vi "Dashboard Main.vi"() -> ()   [LabVIEW 2020]
uses:
  <vilib>/Utility/miscctls.llb/LVRowAndColumnTypeDef.ctl
  <vilib>/event_ctls.llb/eventvkey.ctl
  <vilib>/Rock Robotics/Network Tables/NT Read Numeric Array.vi
  <vilib>/Rock Robotics/WPI/Dashboard/WPI_DashboardLogging Global.vi
panel:
  out "x":dbl(slide) scale=-1.0..1.0 scale format="%#_2e"
  in  "Camera Settings Right":T1={"Frame Rate"=30, "Compression"=30, "Size"=1, "DB Camera Config"=FALSE} {"Frame Rate" scale=1.0..30.0; "Compression" scale=100.0..-1.0; "Size" items=["640x480", "320x240", "160x120"]}
  in  "Camera Name Right":string(combo)="No Camera Selection"
  out "Camera Perf":string
  in  "Camera Settings":T1={"Frame Rate"=30, "Compression"=30, "Size"=1, "DB Camera Config"=FALSE} {"Frame Rate" scale=1.0..30.0; "Compression" scale=100.0..-1.0; "Size" items=["640x480", "320x240", "160x120"]}
  in  "TCP":refnum<k5>
  in  "Rec Mode":enum32{"Stop", "Record", "Playback"}(radio)
  out "Robot IP":string
  out "Image Message":string="Timeout in Camera Communications"
  in  "Dashboard Tab":T2(tab)
  in  "Select Auto":string(combo)="Select Autonomous ..."
  out "NT Connection":bool
  out "MotorChart R":cluster{"Numeric":dbl, "Numeric":dbl}(graph)
  out "MotorChart L":cluster{"Numeric":dbl, "Numeric":dbl}(graph)
  out "MotorSliders R":cluster{"MotorSlide1":dbl, "MotorSlide2":dbl} {"MotorSlide2" scale=-1.0..1.0 scale format="%#_2e"; "MotorSlide1" scale=-1.0..1.0 scale format="%#_2e"}
  out "MotorSliders L":cluster{"MotorSlide1":dbl, "MotorSlide2":dbl} {"MotorSlide2" scale=-1.0..1.0 scale format="%#_2e"; "MotorSlide1" scale=-1.0..1.0 scale format="%#_2e"}
  out "Gyro":dbl(knob) scale=0.0..360.0
  out "JS1 Z":dbl(slide) scale=-1.0..1.0 scale format="%#_2e"
  out "JS1 Graph":cluster{"X":dbl, "Y":dbl}[](graph)
  out "JS1 Buttons":T3
  out "JS2 Z":dbl(slide) scale=-1.0..1.0 scale format="%#_2e"
  out "JS2 Graph":cluster{"X":dbl, "Y":dbl}[](graph)
  out "JS2 Buttons":T3
  out "Mode":T4(ring)=enum."Auto Disabled"
  out "Right Camera Perf":cluster{"Bandwidth (Mbps)":dbl, "FPS":dbl}
  out "Camera Image Right":T5(plugin-control)
  in  "DB/String 9":string
  in  "DB/String 8":string
  in  "DB/String 7":string
  in  "DB/String 6":string
  in  "DB/String 5":string
  in  "DB/String 4":string
  in  "DB/String 3":string
  in  "DB/String 2":string
  in  "DB/String 1":string
  in  "DB/String 0":string
  in  "DB/Slider 0":dbl(slide) scale=0.0..5.0
  in  "DB/Slider 1":dbl(slide) scale=0.0..5.0
  in  "DB/Slider 2":dbl(slide) scale=0.0..5.0
  in  "DB/Slider 3":dbl(slide) scale=0.0..5.0
  out "DB/LED 3":bool
  out "DB/LED 2":bool
  out "DB/LED 1":bool
  out "DB/LED 0":bool
  in  "DB/Button 3":bool
  in  "DB/Button 2":bool
  in  "DB/Button 1":bool
  in  "DB/Button 0":bool caption="New Name"
  in  "Test Slider":dbl(slide) scale=0.0..100.0 scale format="%#_3g"
  in  "On/Off":bool caption="Solenoid"
  in  "Test Name":u16(ring) items=["Select the test to run..."]
  in  "Test Tree":string(tree)
  in  "Motor":cluster{"Value":dbl, "Enable":bool} {"Value" scale=-1.0..1.0 scale format="%#_3g"}
  out "Progress":T6 {"Test Progress" scale=0.0..100.0}
  in  "Rev/Fwd":cluster{"Forward":bool, "Reverse":bool}
  in  "Test Ring":u16(ring) items=["Monochrome", "Color"]
  out "Cmd Status":string
  in  "Execute Command":bool
  in  "Command Params":string[][](table)
  in  "Command Selection":i32(listbox)
  in  "CheckList":i32(listbox)
  out "Tree":string(tree)
  out "Camera Image":T5(plugin-control)
  out "Background":bool
  in  "Camera Name":string(combo)="No Camera Selection"
  # "HW"
  # "HW"
  # "Joysticks"
  # "Drive Motors"
  # "Front"
  # "Right"
  # "Left"
  # "Back"
  # "This tab is a great place for autonomous settings and robot-specific values.\nPlace controls and indicators inside this tab and match name to\nDashboard Variables on robot. You can also delete this comment."
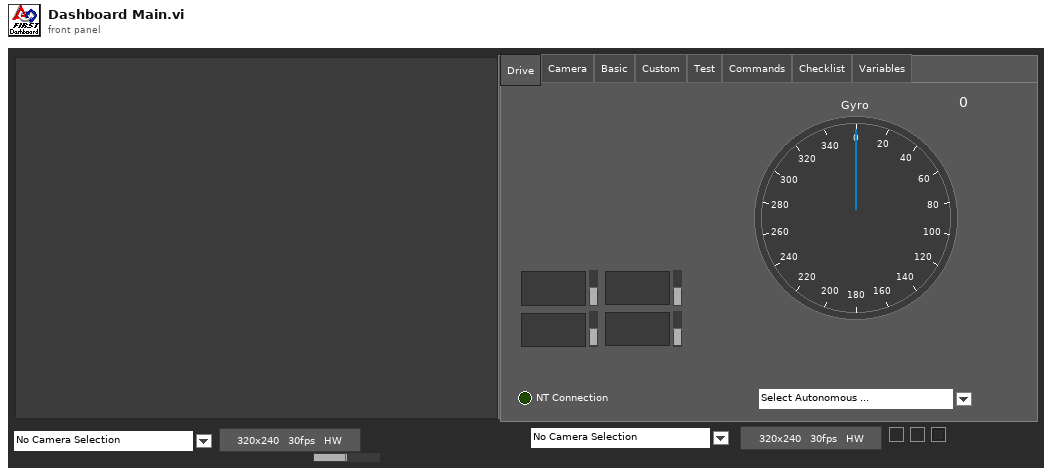
[diagram p1: front panel]
types:
  T1 = cluster{"Frame Rate":i32, "Compression":i32, "Size":u16, "DB Camera Config":bool}
  T2 = enum32{"Drive", "Camera", "Basic", "Custom", "Test", "Commands", "Checklist", "Variables"}
  T3 = cluster{bool, bool, bool, bool, bool, bool, bool, bool, bool, bool, bool, bool}
  T4 = enum8{"Tele-Op Disabled", "Tele-Op Enabled", "Auto Disabled", "Auto Enabled", "Test Disabled", "Test Enabled", "Disconnected", "No Code", "E-Stop"}
  T5 = typedef "IMAQ Image.ctl" = refnum<image>
  T6 = cluster{"Test Progress":u8, "Test Progress Text":string}
  T7 = cluster{"Save Path":path, "Interval (s)":dbl, "Keep":i32}
  T8 = typedef "Image Type" = u32
  T9 = cluster{"IDs":cluster{"RPC field ID":u16, "Unique ID":u16}, "String":string}
  T10 = cluster{"Error Strings":string, "Disable Counts":cluster{u16, u16}, "Rail Faults":cluster{u16, u16, u16}, "Robot IP":string, "DB Mode":u8, "Event Info":cluster{"Name":string, "Type":u8, "Number":u16, "Replay":u8}}
  T11 = cluster{"Storage":cluster{"Disk Free":u64, "RAM Block":u32, "RAM free":u32}, "CPU Utilization":cluster{"CPU % ISR":sgl, "CPU % Time Crit":sgl, "CPU % Timed Str":sgl, "CPU % High":sgl, "CPU % Above":sgl, "CPU % Normal":sgl, "CPU % Low":sgl}, "CAN":cluster{"% Bus Utilization":sgl, "Bus Off Cnt":u32, "TX_FIFO Full Cnt":u32, "Receive Error Cnt":u8, "Transmit Error Cnt":u8}, "HID":cluster{"HID Outputs":u32, "Rumble Low":u16, "Rumble High":u16}[]}
  T12 = cluster{"Status bits":cluster{"Test Mode":bool, "Autonomous":bool, "Enabled":bool, "Code Start":bool, "Brownout":bool, "Reserved 2":bool, "Reserved 3":bool, "E-Stop":bool}, "Code Trace":cluster{"Disabled":bool, "TeleOp":bool, "Auto":bool, "Test":bool}, "Controller Type":enum16{"unknown", "cRIO", "roboRio"}, "Code?":enum16{"unknown", "noCode", "code"}, "Battery V":dbl}
  T13 = cluster{"Control Bits":cluster{"TestMode":bool, "Autonomous":bool, "Enabled":bool, "FMS Present":bool, bool, bool, bool, "E-Stop":bool}, "Team Station ":u8, "Countdown":sgl, "Joystick Values":cluster{"Axes":dbl[], "Buttons":bool[], "POVs":i16[]}[]}
  T14 = cluster{"Axes":dbl[], "Buttons":bool[], "POVs":i16[]}[]
  T15 = cluster{"Axes":dbl[], "Buttons":bool[], "POVs":i16[]}
  T16 = cluster{"Buttons[0]":bool, "Buttons[1]":bool, "Buttons[2]":bool, "Buttons[3]":bool, "Buttons[4]":bool, "Buttons[5]":bool, "Buttons[6]":bool, "Buttons[7]":bool, "Buttons[8]":bool, "Buttons[9]":bool, "Buttons[10]":bool, "Buttons[11]":bool}
  T17 = cluster{"Camera Image":refnum<vi>, "Dashboard Tab":refnum<vi>, "Background":refnum<vi>, "Rec Mode":refnum<vi>, "Test Slider":refnum<vi>, "On/Off ":refnum<vi>, "Test Ring":refnum<vi>, "Rev/Fwd":refnum<vi>, "Test Name":refnum<vi>, "Motor":refnum<vi>, "Progress":refnum<vi>, "CheckList":refnum<vi>, "Tree":refnum<vi>, "Test Tree":refnum<vi>, "Command Params":refnum<vi>, "Command Selection":refnum<vi>, "Execute Command":refnum<vi>, "Cmd Status":refnum<vi>, "Camera Settings":refnum<vi>, "Camera Name":refnum<vi>, "Camera Perf":refnum<vi>, "Camera Settings Right":refnum<vi>, "Camera Name Right":refnum<vi>, "Camera Image Right":refnum<vi>}
  T18 = cluster{"Global Rectangle":i32[], "Contours":cluster{"Contour Type":u32, "ROI Type":u32, "Points":i32[]}[]}
  T19 = cluster{"Camera Name":string, string, "Saved DB Images Info":cluster{"Save Path":path, "Interval (s)":dbl, "Keep":i32}}
  T20 = cluster{"Camera Name Right":string, string, "Saved DB Images Info":cluster{"Save Path":path, "Interval (s)":dbl, "Keep":i32}}
  T21 = cluster{"Operation":enum16{"Update", "Clear"}, "Color Box":u32}[]
  T22 = typedef "eventvkey.ctl" = enum16{"ASCII", "Enter", "Return", "Shift", "Ctrl", "Alt", "Cmd", "Opt", "Caps", "NumLock", "Clear", "Break", "Up", "Down", "Left", "Right", "Insert", "Delete", "Home", "End", "PageUp", "PageDown", "Escape", "Help", "Pause", "ScrollLock", "F1", "F2", "F3", "F4", "F5", "F6", "F7", "F8", "F9", "F10", "F11", "F12", "F13", "F14", "F15", "F16", "F17", "F18", "F19", "F20", "F21", "F22", "F23", "F24", "Play", "VolumeUp", "VolumeDown", "Mute", "Two Byte Char"}
  T23 = cluster{"Image Size":bool, "Image Type":bool, "Pixel Value":bool, "ROI Information":bool, "Zoom Factor":bool}
  T24 = cluster{"Operation":enum16{"Update", "Clear"}, "Color Box":u32}
  T25 = typedef "LVRowAndColumnTypeDef.ctl" = cluster{"Row":i32, "Column":i32}
  T26 = cluster{"Shift":bool, "Ctrl":bool, "Alt":bool, "Cmd":bool, "Opt":bool}
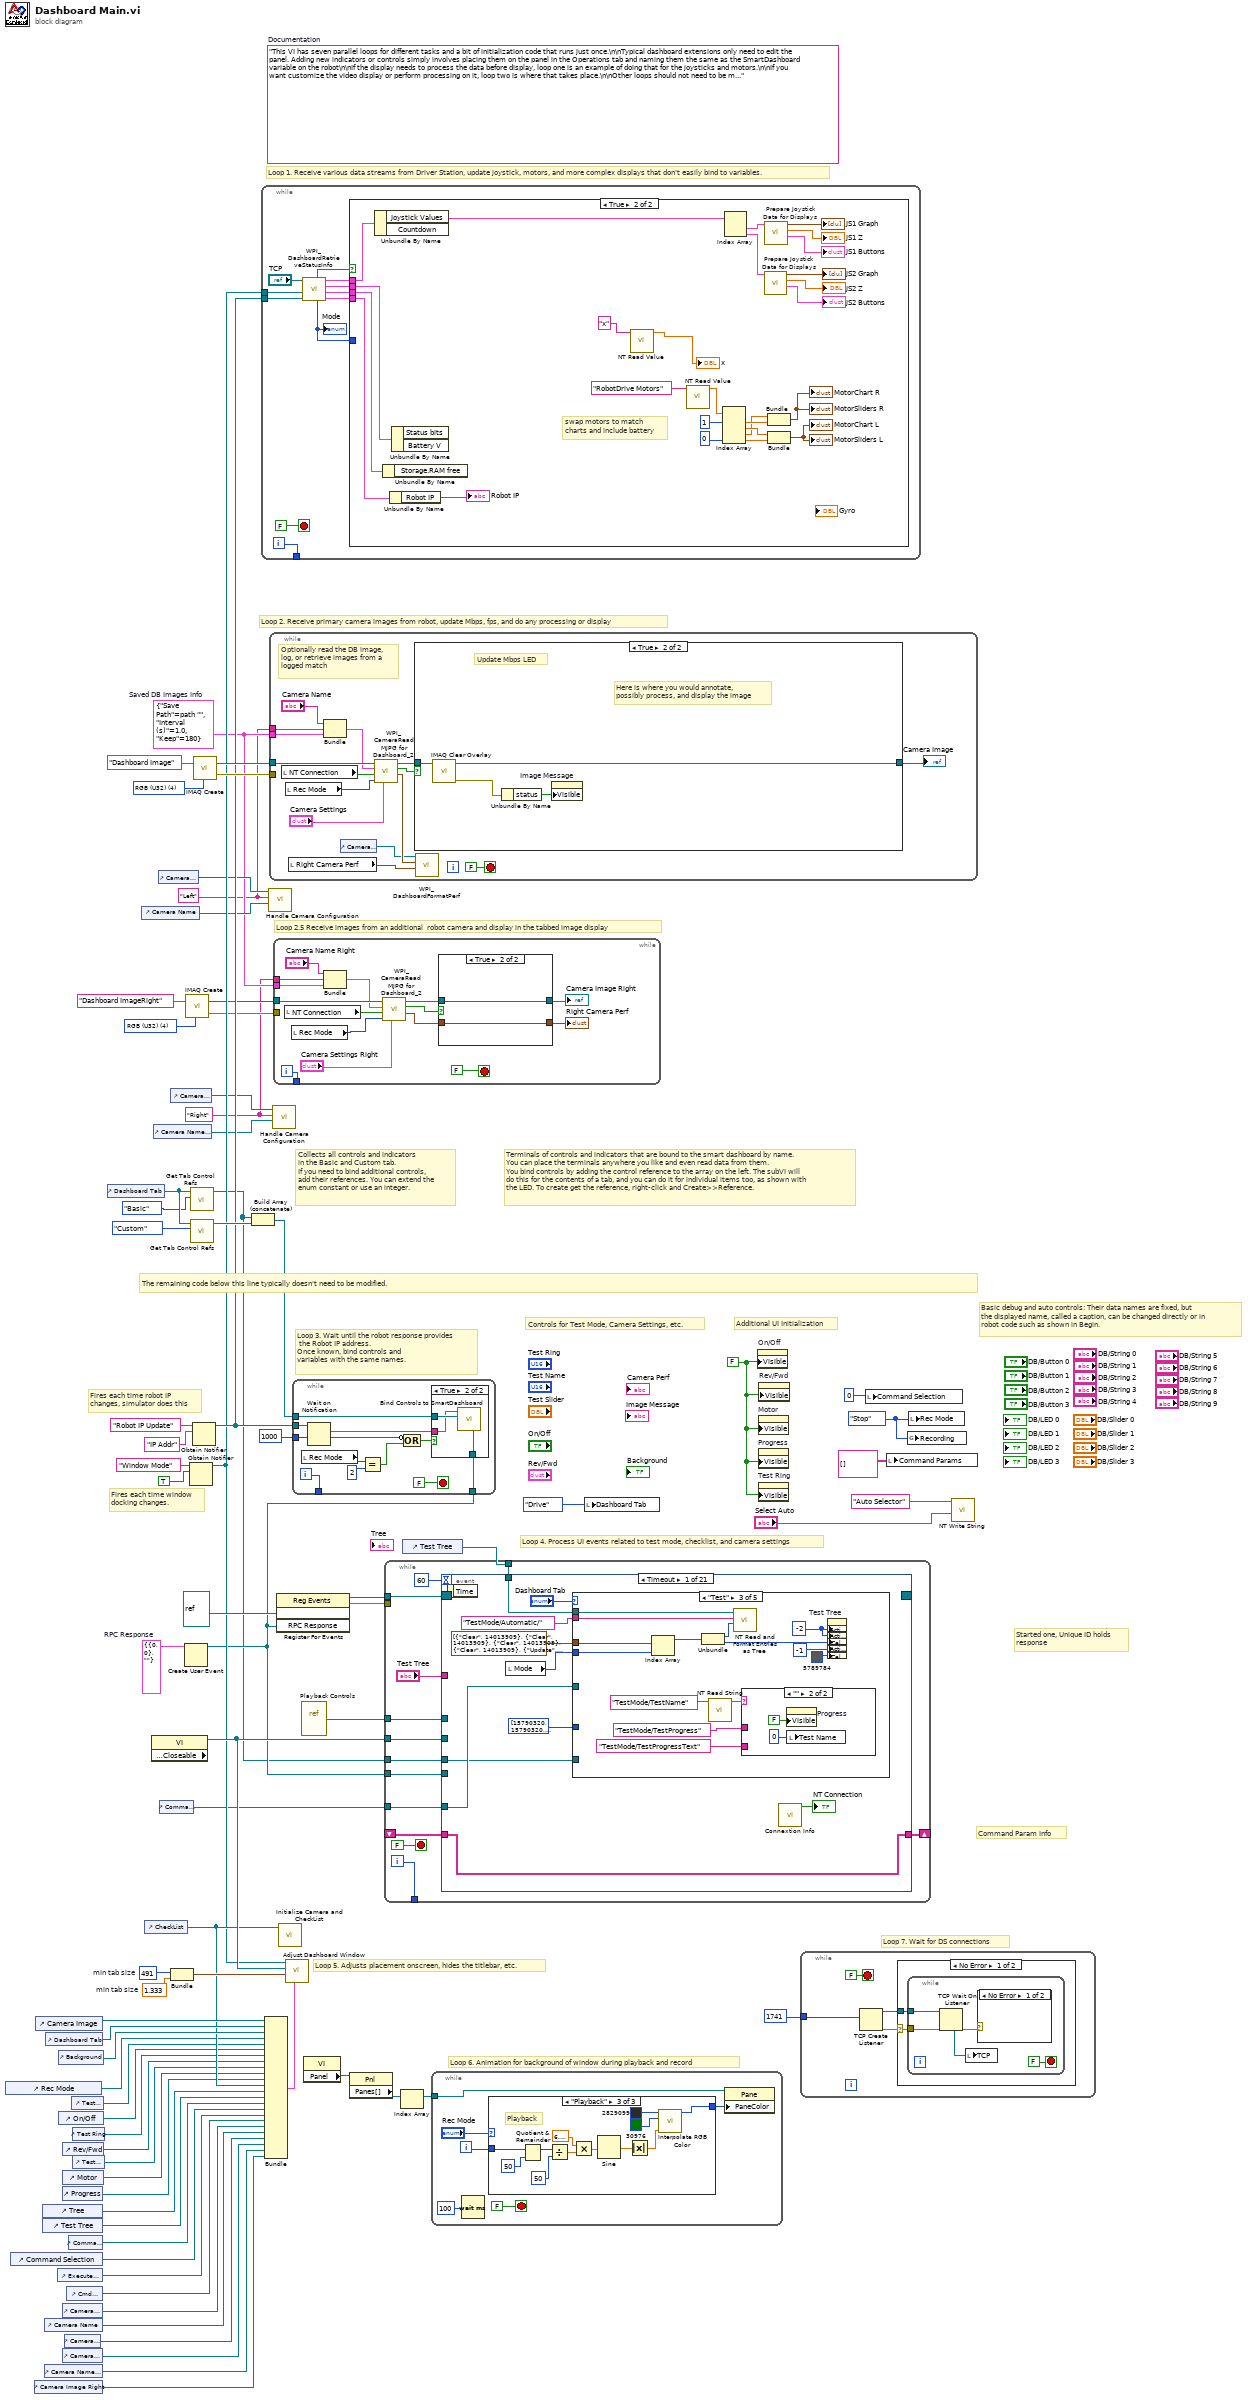
[diagram p0: block diagram]
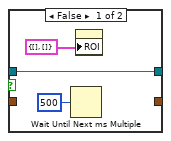
[diagram p2: hidden frame]
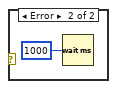
[diagram p3: hidden frame]
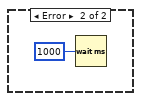
[diagram p4: hidden frame]
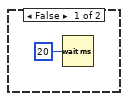
[diagram p5: hidden frame]
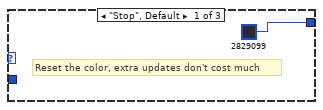
[diagram p6: hidden frame]
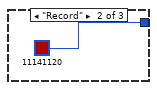
[diagram p7: hidden frame]
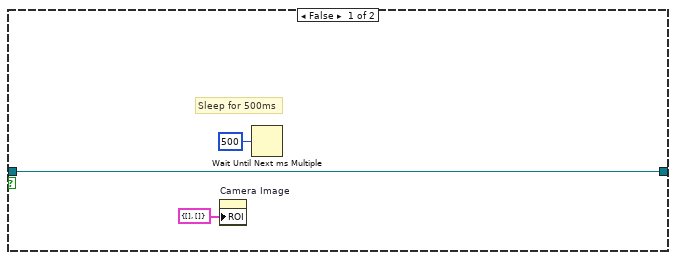
[diagram p9: hidden frame]
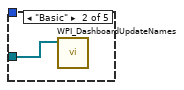
[diagram p11: hidden frame]
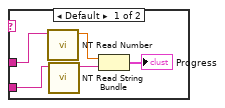
[diagram p12: hidden frame]
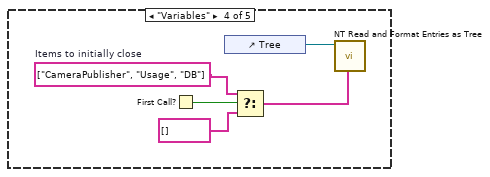
[diagram p13: hidden frame]
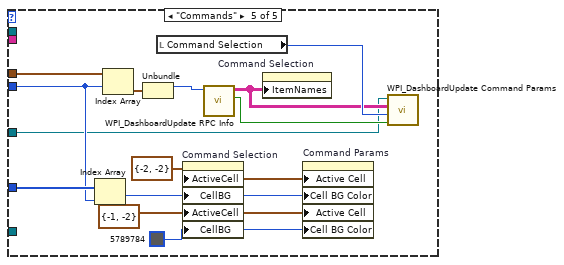
[diagram p14: hidden frame]
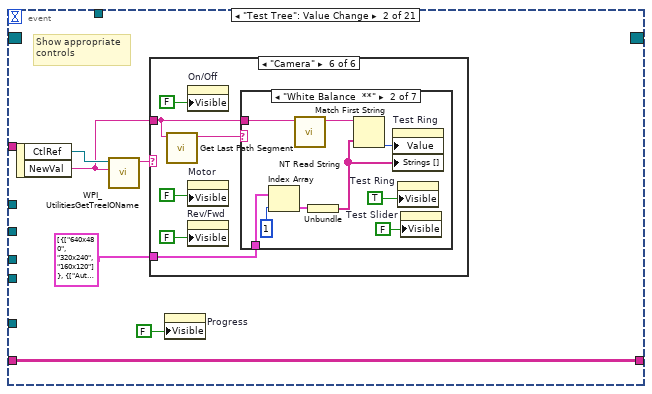
[diagram p15: hidden frame]
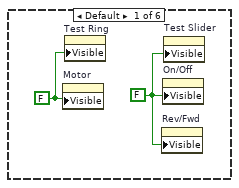
[diagram p16: hidden frame]
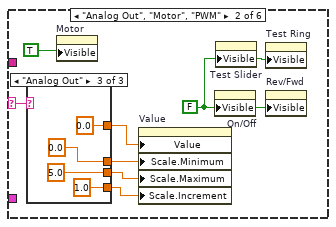
[diagram p17: hidden frame]
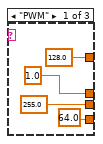
[diagram p18: hidden frame]
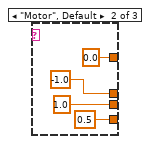
[diagram p19: hidden frame]
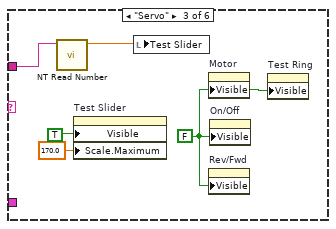
[diagram p20: hidden frame]
diagram:
  w3 = T7 {"Save Path"=path "", "Interval (s)"=1.0, "Keep"=180}  # Saved DB Images Info
  w2 = "Right"
  w1 = "Left"
  w13 = T8 4 items=["Grayscale (U8)", "Grayscale (I16)", "Grayscale (SGL)", "Complex (CSG)", "RGB (U32)", "HSL (U32)", "RGB (U64)"] ("Image Type")
  w29 = T9 {"IDs"={"RPC field ID"=0, "Unique ID"=0}, "String"=""}  # RPC Response
  w52 = 491  # min tab size
  w51 = 1.333  # min tab size
  w59 = enum32{"Stop", "Record", "Playback"}."Stop" ("Rec Mode")
  w36 = FALSE ("Visible")
  (unwired) "This VI has seven parallel loops for different tasks and a bit of initialization code that runs just once.\n\nTypical dashboard extensions only need to edit the panel. Adding new indicators or controls simply involves placing them on the panel in the Operations tab and naming them the same as the SmartDashboard variable on the robot\n\nIf the display needs to process the data before display, loop one is an example of doing that for the joysticks and motors.\n\nIf you want customize the video display or perform processing on it, loop two is where that takes place.\n\nOther loops should not need to be modified. They are pretty standard, and document the task they perform."  # Documentation
  w76 = T8 4 items=["Grayscale (U8)", "Grayscale (I16)", "Grayscale (SGL)", "Complex (CSG)", "RGB (U32)", "HSL (U32)", "RGB (U64)"] ("Image Type")
  # "Loop 2.5 Receive images from an additional  robot camera and display in the tabbed image display"
  # "Command Param Info"
  # "Started one, Unique ID holds\nresponse"
  # "Loop 7. Wait for DS connections"
  # "Basic debug and auto controls: Their data names are fixed, but\nthe displayed name, called a caption, can be changed directly or in\nrobot code such as shown in Begin."
  # "Controls for Test Mode, Camera Settings, etc."
  # "Additional UI Initialization"
  # "Loop 6. Animation for background of window during playback and record"
  # "Fires each time robot IP\nchanges, simulator does this"
  # "Fires each time window\ndocking changes."
  # "Collects all controls and indicators\nin the Basic and Custom tab.\nIf you need to bind additional controls,\nadd their references. You can extend the\nenum constant or use an integer."
  # "The remaining code below this line typically doesn't need to be modified."
  # "Loop 4. Process UI events related to test mode, checklist, and camera settings"
  # "Terminals of controls and indicators that are bound to the smart dashboard by name.\nYou can place the terminals anywhere you like and even read data from them.\nYou bind controls by adding the control reference to the array on the left. The subVI will\ndo this for the contents of a tab, and you can do it for individual items too, as shown with\nthe LED. To create get the reference, right-click and Create>>Reference."
  # "Loop 3. Wait until the robot response provides\n the Robot IP address.\nOnce known, bind controls and\nvariables with the same names."
  # "Loop 5. Adjusts placement onscreen, hides the titlebar, etc."
  # "Loop 1. Receive various data streams from Driver Station, update joystick, motors, and more complex displays that don't easily bind to variables."
  # "Loop 2. Receive primary camera images from robot, update Mbps, fps, and do any processing or display"
  n1 = control-ref of="Rec Mode"() -> (w42:refnum<vi>)
  n2 = control-ref of="Command Selection"() -> (w28:refnum<vi>)
  n3 = control-ref of="Camera Image Right"() -> (w6:refnum<vi>)
  n4 = control-ref of="Camera Image"() -> (w54:refnum<vi>)
  n5 = control-ref of="Tree"() -> (w46:refnum<vi>)
  n6 = control-ref of="Test Tree"() -> (w45:refnum<vi>)
  n7 = control-ref of="Camera Name"() -> (w19:refnum<vi>)
  n8 = control-ref of="Camera Name Right"() -> (w7:refnum<vi>)
  n9 = control-ref of="Dashboard Tab"() -> (w53:refnum<vi>)
  n10 = control-ref of="Execute Command"() -> (w30:refnum<vi>)
  n11 = control-ref of="Background"() -> (w49:refnum<vi>)
  n12 = control-ref of="On/Off"() -> (w40:refnum<vi>)
  n13 = control-ref of="Progress"() -> (w37:refnum<vi>)
  n14 = control-ref of="Camera Settings"() -> (w20:refnum<vi>)
  n15 = control-ref of="Camera Settings Right"() -> (w8:refnum<vi>)
  n16 = control-ref of="Rev/Fwd"() -> (w38:refnum<vi>)
  n17 = control-ref of="Motor"() -> (w43:refnum<vi>)
  n18 = control-ref of="Camera Perf"() -> (w18:refnum<vi>)
  n19 = control-ref of="Cmd Status"() -> (w24:refnum<vi>)
  n20 = control-ref of="Command Params"() -> (w31:refnum<vi>)
  n21 = control-ref of="Test Slider"() -> (w41:refnum<vi>)
  n22 = control-ref of="Test Ring"() -> (w39:refnum<vi>)
  n23 = control-ref of="Test Name"() -> (w44:refnum<vi>)
  n24 = control-ref of="Dashboard Tab"() -> (w57:refnum<vi>)
  n25 = control-ref of="Camera Name"() -> (w21:refnum<vi>)
  n26 = control-ref of="CheckList"() -> (w47:refnum<vi>)
  n27 = property class="VI" props=["Front Panel.Closeable"]() -> (reference out=w58:refnum<vi>)  [unwired: 2 in, 2 out]
  n28 = control-ref of="Camera Name Right"() -> (w9:refnum<vi>)
  n29 = control-ref of="Camera Settings"() -> (w22:refnum<vi>)
  n30 = control-ref of="Command Params"() -> (w23:refnum<vi>)
  n31 = control-ref of="Camera Settings Right"() -> (w10:refnum<vi>)
  n32 = Bundle("min tab size"=w52, "min tab size"=w51) -> (w50:cluster{"min tab size":i32, "min tab size":dbl})  [unwired: 1 in]
  n33 = Create User Event(user event datatype=w29) -> (user event=w25:refnum<user-event>)  [unwired: 1 in, 1 out]
  n34 = call "IMAQ Create"("Image Name"="Dashboard ImageRight", "Image Type"=w13) -> ("New Image"=w12:T5, "error out"=w11:errorcluster)  [unwired: 2 in, 1 out]
  n35 = Obtain Notifier(name (unnamed)="Window Mode", notification data type=TRUE) -> (notifier out=w34:refnum<notifier>)  [unwired: 2 in, 2 out]
  n36 = call <vilib>:"Get Tab Control Refs.vi"("Page Index"=T2."Basic" ("Dashboard Tab"), "TabControl in"=w57) -> ("ControlsOnPage"=w17:refnum<vi>[])  [unwired: 9 in]
  n37 = call <vilib>:"Get Tab Control Refs.vi"("Page Index"=T2."Custom" ("Dashboard Tab"), "TabControl in"=w57) -> ("ControlsOnPage"=w56:refnum<vi>[])  [unwired: 9 in]
  n38 = Obtain Notifier(name (unnamed)="Robot IP Update", notification data type="IP Addr" ("name (unnamed)")) -> (notifier out=w35:refnum<notifier>)  [unwired: 2 in, 2 out]
  n39 = call "IMAQ Create"("Image Name"="Dashboard Image", "Image Type"=w76) -> ("New Image"=w74:T5, "error out"=w73:errorcluster)  [unwired: 2 in, 1 out]
  n40 = Build Array (concatenate)(w17, w56) -> (w55:refnum<vi>[])
  n41 = while {
    tunnel: [w86] -> _
    tunnel: w35 -> [w80]
    tunnel: w34 -> [w77]
    i -> [w86]
    stop <- FALSE stop-if-true
    n42 = call <vilib>:"WPI_DashboardRetrieveStatusInfo.vi"("Binding Refnum"=w80, "Window Mode Notifier"=w77, "TCP Cnx"="TCP") -> ("Power and Errors"=w81:T10, "Robot Metrics"=w84:T11, "Status Info"=w85:T12, "Control Info"=w82:T13, "Robot Mode"=w79:T4, "Process?"=w83:bool)  [unwired: 3 in]
    "Mode" <- w79
    n43 = case shown="True" w83 {
      tunnel: w85 -> [_ w114]
      tunnel: w84 -> [_ w113]
      tunnel: w82 -> [_ w112]
      tunnel: w81 -> [_ w111]
      tunnel: w79 -> [_ _]
      frame False {
        n44 = Wait (ms)(milliseconds to wait=u32 20) -> ()  [unwired: 1 out]
      }
      frame True {
        # "swap motors to match\ncharts and include battery"
        n45 = Unbundle By Name(w112) -> ("Joystick Values"=w102:T14)  [unwired: 1 out]
        n46 = Unbundle By Name(w113) -> ()  [unwired: 1 out]
        n47 = Unbundle By Name(w111) -> ("Robot IP"=→"Robot IP":string)
        n48 = Unbundle By Name(w114) -> ()  [unwired: 2 out]
        n49 = call-poly <vilib>:"NT Read Value.vi"("Name"="x") -> ("Numeric"=→"x":dbl)  [unwired: 9 in, 1 out]
        n50 = call-poly <vilib>:"NT Read Value.vi"("Name"="RobotDrive Motors") -> ("Numeric Array"=w92:dbl[])  [unwired: 9 in, 1 out]
        n51 = Index Array(array=w92, index #1=1, index #4=0) -> (element #1=w106:dbl, element #2=w107:dbl, element #3=w105:dbl, element #4=w110:dbl)  [unwired: 2 in]
        n52 = Index Array(array=w102) -> (element #1=w101:T15, element #2=w97:T15)  [unwired: 2 in]
        n53 = call "Prepare Joystick Data for Displays.vi"("Joystick Values"=w97) -> ("Buttons"=→"JS2 Buttons":T16, "Z Axis"=→"JS2 Z":dbl, "Cartesian Data"=→"JS2 Graph":cluster{"X axis":dbl, "X axis":dbl}[])  [unwired: 8 in]
        n54 = call "Prepare Joystick Data for Displays.vi"("Joystick Values"=w101) -> ("Buttons"=→"JS1 Buttons":T16, "Z Axis"=→"JS1 Z":dbl, "Cartesian Data"=→"JS1 Graph":cluster{"X axis":dbl, "X axis":dbl}[])  [unwired: 8 in]
        n55 = Bundle("Numeric"=w105, "Numeric"=w106) -> (→"MotorChart R" →"MotorSliders R":cluster{"Numeric":dbl, "Numeric":dbl})  [unwired: 1 in]
        n56 = Bundle("Numeric"=w107, "Numeric"=w110) -> (→"MotorChart L" →"MotorSliders L":cluster{"Numeric":dbl, "Numeric":dbl})  [unwired: 1 in]
      }
    }
  }
  n57 = Bundle("Camera Image"=w54, "Dashboard Tab"=w53, "Background"=w49, "Rec Mode"=w42, "Test Slider"=w41, "On/Off"=w40, "Test Ring"=w39, "Rev/Fwd"=w38, "Test Name"=w44, "Motor"=w43, "Progress"=w37, "CheckList"=w47, "Tree"=w46, "Test Tree"=w45, "Command Params"=w31, "Command Selection"=w28, "Execute Command"=w30, "Cmd Status"=w24, "Camera Settings"=w20, "Camera Name"=w19, "Camera Perf"=w18, "Camera Settings Right"=w8, "Camera Name Right"=w7, "Camera Image Right"=w6) -> (w48:T17)  [unwired: 1 in]
  n58 = call "Handle Camera Configuration.vi"("CameraNameRef"=w21, "Display Name"=w1, "ClusterRef"=w22) -> ()  [unwired: 9 in]
  n59 = while {
    tunnel: w74 -> [w128]
    tunnel: w73 -> [_]
    tunnel: w3 -> [w121]
    tunnel: w1 -> [w118]
    stop <- FALSE stop-if-true
    # "Optionally read the DB image,\nlog, or retrieve images from a\nlogged match"
    n60 = local read "NT Connection"() -> (w122:bool)
    n61 = local read "Rec Mode"() -> (w125:enum32{"Stop", "Record", "Playback"})
    n62 = local read "Right Camera Perf"() -> (w116:cluster{"Bandwidth (Mbps)":dbl, "FPS":dbl})
    n63 = Bundle("Camera Name"="Camera Name", w118, "Saved DB Images Info"=w121) -> (w120:T19)  [unwired: 1 in]
    n64 = control-ref of="Camera Perf"() -> (w115:refnum<vi>)
    n65 = call <vilib>:"WPI_CameraRead MJPG for Dashboard_2.vi"("Camera Settings"="Camera Settings", "Rec Mode"=w125, "NT Connection"=w122, "Capture Info"=w120, "Image in"=w128) -> ("perf info"=w117:cluster{"Bandwidth (Mbps)":dbl, "fps":dbl}, "Active"=w126:bool, "Image\\ out"=w127:T5)  [unwired: 4 in]
    n66 = case shown="True" w126 {
      tunnel: w127 -> [w131 w134]
      tunnel: [w131 w133] -> w123
      frame False {
        # "Sleep for 500ms"
        n67 = property on="Camera Image" class="ImageControl"("ROI"=T18 {"Global Rectangle"=[], "Contours"=[]}) -> ()  [unwired: 2 in, 2 out]
        n68 = Wait Until Next ms Multiple(millisecond multiple=u32 500) -> ()  [unwired: 1 out]
      }
      frame True {
        # "Here is where you would annotate,\npossibly process, and display the image"
        # "Update Mbps LED"
        n69 = call "IMAQ Clear Overlay"("Image"=w134) -> ("error out"=w135:errorcluster, "Image Out"=w133:T5)  [unwired: 2 in, 7 out]
        n70 = Unbundle By Name(w135) -> ("status"=w136:bool)
        n71 = property on="Image Message" class="Str"("Visible"=w136) -> ()  [unwired: 2 in, 2 out]
      }
    }
    "Camera Image" <- w123
    n72 = call <vilib>:"WPI_DashboardFormatPerf.vi"("Right Camera Perf"=w116, "Performance"=w117, "String in"=w115) -> ()  [unwired: 9 in]
  }
  n73 = call "Handle Camera Configuration.vi"("CameraNameRef"=w9, "Display Name"=w2, "ClusterRef"=w10) -> ()  [unwired: 9 in]
  n74 = while {
    tunnel: w12 -> [w151]
    tunnel: w11 -> [_]
    tunnel: [w146] -> _
    tunnel: w3 -> [w142]
    tunnel: w2 -> [w139]
    i -> [w146]
    stop <- FALSE stop-if-true
    n75 = local read "NT Connection"() -> (w143:bool)
    n76 = local read "Rec Mode"() -> (w150:enum32{"Stop", "Record", "Playback"})
    n77 = Bundle("Camera Name Right"="Camera Name Right", w139, "Saved DB Images Info"=w142) -> (w141:T20)  [unwired: 1 in]
    n78 = call <vilib>:"WPI_CameraRead MJPG for Dashboard_2.vi"("Camera Settings"="Camera Settings Right", "Rec Mode"=w150, "NT Connection"=w143, "Capture Info"=w141, "Image in"=w151) -> ("perf info"=w137:cluster{"Bandwidth (Mbps)":dbl, "fps":dbl}, "Active"=w145:bool, "Image\\ out"=w148:T5)  [unwired: 4 in]
    n79 = case shown="True" w145 {
      tunnel: w148 -> [w153 w156]
      tunnel: [w153 w156] -> w144
      tunnel: [_ w155] -> w138
      tunnel: w137 -> [_ w155]
      frame False {
        n80 = Wait Until Next ms Multiple(millisecond multiple=u32 500) -> ()  [unwired: 1 out]
        n81 = property on="Camera Image Right" class="ImageControl"("ROI"=T18 {"Global Rectangle"=[], "Contours"=[]}) -> ()  [unwired: 2 in, 2 out]
      }
      frame True {
      }
    }
    "Camera Image Right" <- w144
    "Right Camera Perf" <- w138
  }
  n82 = register-events(refnum<vi> refnum, w25) -> (reference out=w63:refnum<event-registration>, error out=w62:errorcluster)  [unwired: 2 in]
  n83 = call "Initialize Camera and CheckList.vi"("ListBox in"=w47) -> ()  [unwired: 11 in]
  n84 = call "Adjust Dashboard Window.vi"("Sizing Refnums"=w48, "Size Constraints"=w50, "VI"=w58, "WIn Mode"=w34) -> ()  [unwired: 8 in]
  n85 = while {
    tunnel: w55 -> [w168]
    tunnel: w35 -> [w166]
    tunnel: [w164] -> _
    tunnel: u32 1000 ("milliseconds to wait") -> [w163]
    tunnel: w25 -> [w157]
    i -> [w164]
    stop <- FALSE stop-if-true
    n86 = local read "Rec Mode"() -> (w159:enum32{"Stop", "Record", "Playback"})
    n87 = Wait on Notification(notifier=w166, timeout in ms (-1)=w163) -> (notification=w165:string, timed out?=w161:bool)  [unwired: 2 in, 2 out]
    n88 = Equal?(x=w159, y=u16 2 ("Rec Mode")) -> (x = y?=w160:bool)
    n89 = Compound Arithmetic op=OR(invert w161, w160) -> (w162:bool)
    n90 = case shown="True" w162 {
      tunnel: w168 -> [_ w171]
      tunnel: w165 -> [_ w170]
      tunnel: w157 -> [_ w169]
      frame False {
      }
      frame True {
        n91 = call <vilib>:"Bind Controls to SmartDashboard.vi"("RPC ref"=w169, "Bound Control Refs"=w171, "Server IP Address"=w170) -> ()  [unwired: 9 in]
      }
    }
  }
  n92 = vi-ref "Playback Controls.vi"() -> (w64:refnum<vi>)
  n93 = property class="VI"() -> ("Panel"=w66:refnum<vi>)  [unwired: 2 in, 2 out]
  n94 = property class="Pnl"(reference=w66) -> ("Panes[]"=w67:refnum<vi>[])  [unwired: 1 in, 2 out]
  n95 = Index Array(array=w67) -> (element=w65:refnum<vi>)  [unwired: 1 in]
  n96 = control-ref of="Test Tree"() -> (w68:refnum<vi>)
  n97 = while {
    tunnel: [w181] -> _
    tunnel: w68 -> [w180]
    tunnel: w64 -> [w179]
    tunnel: w63 -> [w178]
    tunnel: w62 -> [_]
    tunnel: w58 -> [w177]
    tunnel: w25 -> [w176]
    tunnel: w23 -> [w175]
    shift-right: [w174] -> _
    shift-left: _ -> [w173]
    tunnel: w17 -> [w172]
    i -> [w181]
    stop <- FALSE stop-if-true
    n98 = event shown="[0] Timeout" {
      selector: w178 -> [_ _ _ _ _ _ _ _ _ _ _ _ _ _ _ _ _ _ _ _ _]
      dyn-events: [_ _ _ _ _ _ _ _ _ _ _ _ _ _ _ _ w441 _ _ _ _] -> _
      timeout: u32 60 ("milliseconds to wait") -> [_ _ _ _ _ _ _ _ _ _ _ _ _ _ _ _ _ _ _ _ _]
      tunnel: w180 -> [w193 _ _ _ _ _ _ _ _ _ _ _ _ _ _ _ _ _ _ _ _]
      tunnel: "Test Tree" -> [_ _ _ _ _ _ _ _ _ _ _ w408 w416 w418 w422 w430 _ _ _ _ _]
      tunnel: w179 -> [_ _ _ _ _ _ _ _ _ _ _ _ _ _ _ _ w443 _ w461 _ _]
      tunnel: w177 -> [_ _ _ _ _ _ _ _ _ _ _ _ _ _ _ _ w439 _ _ _ _]
      tunnel: w176 -> [_ _ _ _ _ _ _ _ _ _ _ _ _ _ _ _ w437 _ _ _ _]
      tunnel: w175 -> [w188 _ _ _ _ _ w359 _ _ _ _ _ _ _ _ _ _ _ _ _ _]
      tunnel: [w187 w236 w338 w343 w352 w356 w357 w366 w376 w383 w395 w407 w414 w417 w421 w429 w436 w456 w458 w462 w475] -> w174
      tunnel: w173 -> [w187 w236 w338 w343 w352 w356 w357 _ _ w383 w395 w407 w414 w417 w421 w429 w436 w456 w458 w462 w475]
      tunnel: w172 -> [w185 _ _ _ _ _ _ _ _ _ _ _ _ _ _ _ _ _ _ _ _]
      event Timeout {
        n99 = event-data() -> ()  [unwired: 1 in, 1 out]
        n100 = local read "Mode"() -> (w190:T4)
        n101 = case shown="\"Test\"" "Dashboard Tab" {
          tunnel: w193 -> [_ _ w209 _ _]
          tunnel: "TestMode/Automatic/" ("Name Pattern") -> [_ _ w208 _ _]
          tunnel: T21 [{"Operation"=enum."Clear", "Color Box"=14013909}, {"Operation"=enum."Clear", "Color Box"=14013909}, {"Operation"=enum."Clear", "Color Box"=14013909}, {"Operation"=enum."Clear", "Color Box"=14013909}, {"Operation"=enum."Update", "Color Box"=14013909}, {"Operation"=enum."Update", "Color Box"=16777215}, {"Operation"=enum."Clear", "Color Box"=14013909}, {"Operation"=enum."Clear", "Color Box"=14013909}, {"Operation"=enum."Clear", "Color Box"=14013909}] -> [_ _ w201 _ w229]
          tunnel: w190 -> [_ _ w200 _ w228]
          tunnel: u32[] [15790320, 15790320, 15790320, 15790320, 16777215, 16777215, 15790320, 15790320, 15790320] -> [_ _ _ _ w234]
          tunnel: w188 -> [_ _ _ _ w222]
          tunnel: w185 -> [_ w195 _ _ _]
          frame "Custom", Default {
          }
          frame "Basic" {
            n102 = call <vilib>:"WPI_DashboardUpdateNames.vi"("Controls on Tab"=w195) -> ()  [unwired: 11 in]
          }
          frame "Test" {
            w207 = -2 ("Active Item:Row Number")
            n103 = Index Array(array=w201, index=w200) -> (element=w202:T24)
            n104 = Unbundle(w202) -> ("Operation"=w203:enum16{"Update", "Clear"}, "Color Box"=w204:u32)
            n105 = call <vilib>:"NT Read String.vi"("Name"="TestMode/TestName") -> ("String"=w198:string)  [unwired: 9 in, 1 out]
            n106 = call <vilib>:"NT Read and Format Entries as Tree.vi"("Operation"=w203, "Name Pattern"=w208, "Tree Refnum"=w209) -> ()  [unwired: 7 in, 2 out]
            n107 = case shown="\"\"" w198 {
              tunnel: "TestMode/TestProgress" ("Name") -> [w211 _]
              tunnel: "TestMode/TestProgressText" ("Name") -> [w210 _]
              frame Default {
                n108 = call <vilib>:"NT Read Number.vi"("Name"=w211) -> ("Numeric"=w212:dbl)  [unwired: 9 in, 1 out]
                n109 = call <vilib>:"NT Read String.vi"("Name"=w210) -> ("String"=w213:string)  [unwired: 9 in, 1 out]
                n110 = Bundle("Numeric"=w212, "String"=w213) -> (→"Progress":cluster{"Numeric":dbl, "String":string})  [unwired: 1 in]
              }
              frame "" {
                n111 = property on="Progress" class="Clust (strict)"("Visible"=FALSE) -> ()  [unwired: 2 in, 2 out]
                n112 = local write "Test Name"(u16 0) -> ()
              }
            }
            n113 = property on="Test Tree" class="Tree (strict)"("Active Item Row Number"=w207, "ActiveColNum"=w207, "CellBG"=w204, "Active Item Row Number"=-1 ("Active Item:Row Number"), "CellBG"=u32 5789784 ("Color Box")) -> ()  [unwired: 2 in, 2 out]
          }
          frame "Variables" {
            w219 = string[] ["CameraPublisher", "Usage", "DB"]  # Items to initially close
            n114 = First Call?() -> (First Call?: T/F=w220:bool)
            n115 = control-ref of="Tree"() -> (w221:refnum<vi>)
            n116 = Select(t=w219, s=w220, f=string[] []) -> (s? t:f=w217:string[])
            n117 = call <vilib>:"NT Read and Format Entries as Tree.vi"("Tags to  Close"=w217, "Tree Refnum"=w221) -> ()  [unwired: 8 in, 2 out]
          }
          frame "Commands" {
            w230 = u32 5789784 ("Color Box")
            w231 = T25 {"Row"=-1, "Column"=-2} ("Active Cell:Active Cell")
            w233 = T25 {"Row"=-2, "Column"=-2} ("Active Cell:Active Cell")
            n118 = Index Array(array=w234, index=w228) -> (element=w232:u32)
            n119 = Index Array(array=w229, index=w228) -> (element=w227:T24)
            n120 = Unbundle(w227) -> ("Operation"=w226:enum16{"Update", "Clear"})  [unwired: 1 out]
            n121 = local read "Command Selection"() -> (w225:i32)
            n122 = property on="Command Selection" class="MCListbox (strict)"("ActiveCell"=w233, "CellBG"=w232, "ActiveCell"=w231, "CellBG"=w230) -> ()  [unwired: 2 in, 2 out]
            n123 = call <vilib>:"WPI_DashboardUpdate RPC Info.vi"("Operation"=w226) -> ("update"=w224:bool, "commands"=w223:string[][])  [unwired: 9 in]
            n124 = property on="Command Selection" class="MCListbox (strict)"("ItemNames"=w223) -> ()  [unwired: 2 in, 2 out]
            n125 = property on="Command Params" class="Tbl (strict)"("Active Cell"=w233, "Cell BG Color"=w232, "Active Cell"=w231, "Cell BG Color"=w230) -> ()  [unwired: 2 in, 2 out]
            n126 = call <vilib>:"WPI_DashboardUpdate Command Params.vi"("Update"=w224, "NewVal"=w225, "Commands"=w223, "Param Tbl"=w222) -> ()  [unwired: 7 in, 1 out]
          }
        }
        n127 = call <vilib>:"Connextion Info.vi"() -> ("Connected"=→"NT Connection":bool)  [unwired: 10 in, 1 out]
      }
      event "Test Tree": Value Change {
        # "Show appropriate\ncontrols"
        n128 = event-data() -> ("CtlRef"=w239:refnum<vi>, "NewVal"=w237:string)  [unwired: 1 in]
        n129 = call <vilib>:"WPI_UtilitiesGetTreeIOName.vi"("NewVal"=w237, "TreeControl in"=w239) -> ("I/O Name"=w240:string)  [unwired: 9 in]
        n130 = case shown="\"Camera\"" w240 {
          selector: w240 -> [_ w247 _ w269 w278 _]
          tunnel: w237 -> [_ _ w266 w268 _ w285]
          tunnel: cluster{string[]}[] [{["640x480", "320x240", "160x120"]}, {["Auto", "Fixed indoor", "Fixed outdoor 1", "Fixed outdoor 2", "Fixed fluorescent 1", "Fixed fluorescent 2", "Hold current"]}, {["Auto", "Flicker-free 50 Hz", "Flicker-free 60 Hz", "Hold current"]}, {["None", "Prioritize frame rate", "Prioritize image quality"]}, {["Monochrome", "Color"]}] -> [_ _ _ _ _ w284]
          frame Default {
            w242 = FALSE ("Visible")
            w241 = FALSE ("Visible")
            n131 = property on="Motor" class="Clust (strict)"("Visible"=w241) -> ()  [unwired: 2 in, 2 out]
            n132 = property on="Test Ring" class="Ring (strict)"("Visible"=w241) -> ()  [unwired: 2 in, 2 out]
            n133 = property on="Rev/Fwd" class="Clust (strict)"("Visible"=w242) -> ()  [unwired: 2 in, 2 out]
            n134 = property on="On/Off" class="Bool (strict)"("Visible"=w242) -> ()  [unwired: 2 in, 2 out]
            n135 = property on="Test Slider" class="Slide (strict)"("Visible"=w242) -> ()  [unwired: 2 in, 2 out]
          }
          frame "Analog Out", "Motor", "PWM" {
            w248 = FALSE ("Visible")
            n136 = case shown="\"Analog Out\"" w247 {
              tunnel: [1.0 ("Value") -1.0 ("Value") 0.0 ("Value")] -> w246
              tunnel: [255.0 ("Value") 1.0 ("Value") 5.0 ("Value")] -> w245
              tunnel: [128.0 ("Value") 0.0 ("Value") 0.0 ("Value")] -> w244
              tunnel: [64.0 ("Value") 0.5 ("Value") 1.0 ("Value")] -> w243
              frame "PWM" {
              }
              frame "Motor", Default {
              }
              frame "Analog Out" {
              }
            }
            n137 = property on="Motor" class="Clust (strict)"("Visible"=TRUE) -> ()  [unwired: 2 in, 2 out]
            n138 = property on="Value" class="Slide (strict)"("Value"=w244, "Scale.Minimum"=w246, "Scale.Maximum"=w245, "Scale.Increment"=w243) -> ()  [unwired: 2 in, 2 out]
            n139 = property on="On/Off" class="Bool (strict)"("Visible"=w248) -> ()  [unwired: 2 in, 2 out]
            n140 = property on="Test Slider" class="Slide (strict)"("Visible"=w248) -> ()  [unwired: 2 in, 2 out]
            n141 = property on="Test Ring" class="Ring (strict)"("Visible"=w248) -> ()  [unwired: 2 in, 2 out]
            n142 = property on="Rev/Fwd" class="Clust (strict)"("Visible"=w248) -> ()  [unwired: 2 in, 2 out]
          }
          frame "Servo" {
            w264 = FALSE ("Visible")
            n143 = call <vilib>:"NT Read Number.vi"("Name"=w266) -> ("Numeric"=w265:dbl)  [unwired: 9 in, 1 out]
            n144 = property on="Test Slider" class="Slide (strict)"("Visible"=TRUE, "Scale.Maximum"=170.0 ("Scale.Range:Maximum")) -> ()  [unwired: 2 in, 2 out]
            n145 = local write "Test Slider"(w265) -> ()
            n146 = property on="Motor" class="Clust (strict)"("Visible"=w264) -> ()  [unwired: 2 in, 2 out]
            n147 = property on="Rev/Fwd" class="Clust (strict)"("Visible"=w264) -> ()  [unwired: 2 in, 2 out]
            n148 = property on="On/Off" class="Bool (strict)"("Visible"=w264) -> ()  [unwired: 2 in, 2 out]
            n149 = property on="Test Ring" class="Ring (strict)"("Visible"=w264) -> ()  [unwired: 2 in, 2 out]
          }
          frame "Relay", "Solenoid" {
            w267 = FALSE ("Visible")
            n150 = property on="Motor" class="Clust (strict)"("Visible"=w267) -> ()  [unwired: 2 in, 2 out]
            n151 = property on="Test Slider" class="Slide (strict)"("Visible"=w267) -> ()  [unwired: 2 in, 2 out]
            n152 = Search and Replace String(input string=w268, search string="/Value  **", replace string="/Direction") -> (result string=w274:string)  [unwired: 5 in, 3 out]
            n153 = property on="Test Ring" class="Ring (strict)"("Visible"=w267) -> ()  [unwired: 2 in, 2 out]
            n154 = call <vilib>:"NT Read String.vi"("Name"=w274) -> ("String"=w272:string)  [unwired: 9 in, 1 out]
            n155 = Equal?(x="Both directions", y=w272) -> (x = y?=w270:bool)
            n156 = Not(x=w270) -> (.not. x?=w271:bool)
            n157 = property on="Rev/Fwd" class="Clust (strict)"("Visible"=w270) -> ()  [unwired: 2 in, 2 out]
            n158 = property on="On/Off" class="Bool (strict)"("Visible"=w271, "Caption.Text"=w269) -> ()  [unwired: 2 in, 2 out]
          }
          frame "Compressor", "Digital Out" {
            w277 = FALSE ("Visible")
            # "Get direction and finish"
            n159 = property on="Motor" class="Clust (strict)"("Visible"=w277) -> ()  [unwired: 2 in, 2 out]
            n160 = property on="Test Slider" class="Slide (strict)"("Visible"=w277) -> ()  [unwired: 2 in, 2 out]
            n161 = property on="Test Ring" class="Ring (strict)"("Visible"=w277) -> ()  [unwired: 2 in, 2 out]
            n162 = property on="On/Off" class="Bool (strict)"("Visible"=TRUE, "Caption.Text"=w278) -> ()  [unwired: 2 in, 2 out]
            n163 = property on="Rev/Fwd" class="Clust (strict)"("Visible"=FALSE) -> ()  [unwired: 2 in, 2 out]
          }
          frame "Camera" {
            n164 = call <vilib>:"Get Last Path Segment.vi"("String in"=w285) -> ("String out"=w286:string)  [unwired: 10 in]
            n165 = property on="On/Off" class="Bool (strict)"("Visible"=FALSE) -> ()  [unwired: 2 in, 2 out]
            n166 = property on="Motor" class="Clust (strict)"("Visible"=FALSE) -> ()  [unwired: 2 in, 2 out]
            n167 = property on="Rev/Fwd" class="Clust (strict)"("Visible"=FALSE) -> ()  [unwired: 2 in, 2 out]
            n168 = case shown="\"White Balance  **\"" w286 {
              tunnel: w285 -> [w292 w301 w310 w319 w328 _ w334]
              tunnel: w284 -> [w290 w298 w307 w316 w325 _ _]
              frame "Size  **" {
                n169 = Index Array(array=w290) -> (element=w289:cluster{string[]})  [unwired: 1 in]
                n170 = call <vilib>:"NT Read String.vi"("Name"=w292) -> ("String"=w291:string)  [unwired: 9 in, 1 out]
                n171 = Unbundle(w289) -> (w287:string[])
                n172 = Match First String(2:w287, 3:w291) -> (0:w288:i32)  [unwired: 1 out]
                n173 = property on="Test Ring" class="Ring (strict)"("Value"=w288, "Strings []"=w287) -> ()  [unwired: 2 in, 2 out]
                n174 = property on="Test Ring" class="Ring (strict)"("Visible"=TRUE) -> ()  [unwired: 2 in, 2 out]
                n175 = property on="Test Slider" class="Slide (strict)"("Visible"=FALSE) -> ()  [unwired: 2 in, 2 out]
              }
              frame "White Balance  **" {
                n176 = Index Array(array=w298, index=1) -> (element=w299:cluster{string[]})
                n177 = call <vilib>:"NT Read String.vi"("Name"=w301) -> ("String"=w300:string)  [unwired: 9 in, 1 out]
                n178 = Unbundle(w299) -> (w296:string[])
                n179 = Match First String(2:w296, 3:w300) -> (0:w295:i32)  [unwired: 1 out]
                n180 = property on="Test Ring" class="Ring (strict)"("Value"=w295, "Strings []"=w296) -> ()  [unwired: 2 in, 2 out]
                n181 = property on="Test Ring" class="Ring (strict)"("Visible"=TRUE) -> ()  [unwired: 2 in, 2 out]
                n182 = property on="Test Slider" class="Slide (strict)"("Visible"=FALSE) -> ()  [unwired: 2 in, 2 out]
              }
              frame "Exposure  **" {
                n183 = Index Array(array=w307, index=2) -> (element=w308:cluster{string[]})
                n184 = call <vilib>:"NT Read String.vi"("Name"=w310) -> ("String"=w309:string)  [unwired: 9 in, 1 out]
                n185 = Unbundle(w308) -> (w304:string[])
                n186 = Match First String(2:w304, 3:w309) -> (0:w305:i32)  [unwired: 1 out]
                n187 = property on="Test Ring" class="Ring (strict)"("Value"=w305, "Strings []"=w304) -> ()  [unwired: 2 in, 2 out]
                n188 = property on="Test Ring" class="Ring (strict)"("Visible"=TRUE) -> ()  [unwired: 2 in, 2 out]
                n189 = property on="Test Slider" class="Slide (strict)"("Visible"=FALSE) -> ()  [unwired: 2 in, 2 out]
              }
              frame "Exposure Priority  **" {
                n190 = Index Array(array=w316, index=3) -> (element=w317:cluster{string[]})
                n191 = call <vilib>:"NT Read String.vi"("Name"=w319) -> ("String"=w318:string)  [unwired: 9 in, 1 out]
                n192 = Unbundle(w317) -> (w313:string[])
                n193 = Match First String(2:w313, 3:w318) -> (0:w314:i32)  [unwired: 1 out]
                n194 = property on="Test Ring" class="Ring (strict)"("Value"=w314, "Strings []"=w313) -> ()  [unwired: 2 in, 2 out]
                n195 = property on="Test Ring" class="Ring (strict)"("Visible"=TRUE) -> ()  [unwired: 2 in, 2 out]
                n196 = property on="Test Slider" class="Slide (strict)"("Visible"=FALSE) -> ()  [unwired: 2 in, 2 out]
              }
              frame "Color Enable  **" {
                n197 = Index Array(array=w325, index=4) -> (element=w326:cluster{string[]})
                n198 = call <vilib>:"NT Read String.vi"("Name"=w328) -> ("String"=w327:string)  [unwired: 9 in, 1 out]
                n199 = Unbundle(w326) -> (w322:string[])
                n200 = Match First String(2:w322, 3:w327) -> (0:w323:i32)  [unwired: 1 out]
                n201 = property on="Test Ring" class="Ring (strict)"("Value"=w323, "Strings []"=w322) -> ()  [unwired: 2 in, 2 out]
                n202 = property on="Test Ring" class="Ring (strict)"("Visible"=TRUE) -> ()  [unwired: 2 in, 2 out]
                n203 = property on="Test Slider" class="Slide (strict)"("Visible"=FALSE) -> ()  [unwired: 2 in, 2 out]
              }
              frame Default {
                n204 = property on="Test Ring" class="Ring (strict)"("Visible"=FALSE) -> ()  [unwired: 2 in, 2 out]
                n205 = property on="Test Slider" class="Slide (strict)"("Visible"=FALSE) -> ()  [unwired: 2 in, 2 out]
              }
              frame "Brightness  **", "Color Level  **", "Compression  **", "FPS  **", "Sharpness  **" {
                n206 = call <vilib>:"NT Read Number.vi"("Name"=w334) -> ("Numeric"=w333:dbl)  [unwired: 9 in, 1 out]
                n207 = local write "Test Slider"(w333) -> ()
                n208 = property on="Test Slider" class="Slide (strict)"("Visible"=TRUE, "Scale.Maximum"=100.0 ("Scale.Range:Maximum")) -> ()  [unwired: 2 in, 2 out]
                n209 = property on="Test Ring" class="Ring (strict)"("Visible"=FALSE) -> ()  [unwired: 2 in, 2 out]
              }
            }
          }
        }
        n210 = property on="Progress" class="Clust (strict)"("Visible"=FALSE) -> ()  [unwired: 2 in, 2 out]
      }
      event "Test Name": Mouse Enter {
        # "Populate the ring with the list of tests"
        n211 = event-data() -> ()  [unwired: 1 in, 1 out]
        n212 = call <vilib>:"NT Read String Array.vi"("Name"="TestMode/TestList") -> ("String Array"=w342:string[])  [unwired: 9 in, 1 out]
        n213 = Build Array (concatenate)("Select the test to run...", w342) -> (w341:string[])
        n214 = property on="Test Name" class="Ring (strict)"("Strings []"=w341) -> ()  [unwired: 2 in, 2 out]
      }
      event "Test Name": Value Change {
        w344 = FALSE ("Visible")
        # "Tell the robot the test name to run"
        n215 = event-data() -> ("NewVal"=w348:u16)  [unwired: 1 in]
        n216 = property on="Test Name" class="Ring (strict)"() -> ("Strings []"=w349:string[])  [unwired: 2 in, 2 out]
        n217 = local write "Progress"(T6 {"Test Progress"=0, "Test Progress Text"=""} ("Progress")) -> ()
        n218 = Index Array(array=w349, index=w348) -> (element=w347:string)
        n219 = call <vilib>:"NT Write String.vi"("String"=w347, "Name"="TestMode/TestName") -> ()  [unwired: 9 in, 1 out]
        n220 = property on="Progress" class="Clust (strict)"("Visible"=TRUE) -> ()  [unwired: 2 in, 2 out]
        n221 = property on="Motor" class="Clust (strict)"("Visible"=w344) -> ()  [unwired: 2 in, 2 out]
        n222 = property on="Test Slider" class="Slide (strict)"("Visible"=w344) -> ()  [unwired: 2 in, 2 out]
        n223 = property on="On/Off" class="Bool (strict)"("Visible"=w344) -> ()  [unwired: 2 in, 2 out]
        n224 = property on="Rev/Fwd" class="Clust (strict)"("Visible"=w344) -> ()  [unwired: 2 in, 2 out]
        n225 = property on="Test Ring" class="Ring (strict)"("Visible"=w344) -> ()  [unwired: 2 in, 2 out]
      }
      event "Select Auto": Mouse Enter {
        # "Populate the combo box with the list of autonomous options"
        n226 = event-data() -> ()  [unwired: 1 in, 1 out]
        n227 = call <vilib>:"NT Read String Array.vi"("Name"="Auto List") -> ("String Array"=w351:string[])  [unwired: 9 in, 1 out]
        n228 = property on="Select Auto" class="CmbBox"("Strings[]"=w351) -> ()  [unwired: 2 in, 2 out]
      }
      event "Select Auto": Value Change {
        # "User modified the Auto Selection. Write to NT variable so robot knows."
        n229 = event-data() -> ("NewVal"=w354:string)  [unwired: 1 in]
        n230 = call <vilib>:"NT Write String.vi"("String"=w354, "Name"="Auto Selector") -> ()  [unwired: 9 in, 1 out]
      }
      event "Command Selection": Value Change {
        # "Get the params and show in table"
        n231 = event-data() -> ("NewVal"=w360:i32)  [unwired: 1 in]
        n232 = property on="Command Selection" class="MCListbox (strict)"() -> ("ItemNames"=w358:string[][])  [unwired: 2 in, 2 out]
        n233 = call <vilib>:"WPI_DashboardUpdate Command Params.vi"("NewVal"=w360, "Commands"=w358, "Param Tbl"=w359) -> ()  [unwired: 8 in, 1 out]
      }
      event "Execute Command": Value Change {
        # "Started one, Unique ID holds\nresponse"
        n234 = event-data() -> ()  [unwired: 1 in, 1 out]
        n235 = property on="Command Selection" class="MCListbox (strict)"() -> ("ItemNames"=w371:string[][])  [unwired: 2 in, 2 out]
        n236 = Index Array(array=w371, index (row)="Command Selection", index (col)=0) -> (element=w369:string)
        n237 = call <vilib>:"Invoke Commands.vi"("Command Params"="Command Params", "Function Name"=w369) -> ("Params"=w365:u8, "Started"=w364:bool)  [unwired: 7 in, 1 out]
        n238 = Array Subset(array="Command Params", length (row)=w365) -> (w366:string[][])  [unwired: 3 in]
        n239 = Select(t="Executing" ("Cmd Status"), s=w364, f="" ("Cmd Status")) -> (s? t:f=→"Cmd Status":string)
      }
      event "Command Selection": Double Click {
        n240 = event-data() -> ("Row"=w379:i32)  [unwired: 1 in]
        n241 = property on="Command Selection" class="MCListbox (strict)"() -> ("ItemNames"=w382:string[][])  [unwired: 2 in, 2 out]
        n242 = local read "Command Params"() -> (w378:string[][])
        n243 = Index Array(array=w382, index (row)=w379, index (col)=0) -> (element=w380:string)
        n244 = call <vilib>:"Invoke Commands.vi"("Command Params"=w378, "Function Name"=w380) -> ("Params"=w377:u8, "Started"=w372:bool)  [unwired: 7 in, 1 out]
        n245 = Array Subset(array=w378, length (row)=w377) -> (w376:string[][])  [unwired: 3 in]
        n246 = Select(t="Executing" ("Cmd Status"), s=w372, f="" ("Cmd Status")) -> (s? t:f=w373:string)
        n247 = local write "Cmd Status"(w373) -> ()
      }
      event "CheckList": Double Click {
        # "Shift clears all"
        # "Update symbols on the listbox"
        n248 = event-data() -> ("PlatMods.Shift"=w384:bool, "Row"=w386:i32)  [unwired: 1 in]
        n249 = case shown="True" w384 {
          tunnel: w386 -> [w390 _]
          tunnel: 1 -> [w389 _]
          frame False {
            n250 = property on="CheckList" class="LstBox (strict)"() -> ("Item Symbols"=w388:i32[])  [unwired: 2 in, 2 out]
            n251 = Replace Array Subset(array=w388, new element=w389, index=w390) -> (w387:i32[])
            n252 = property on="CheckList" class="LstBox (strict)"("Item Symbols"=w387) -> ()  [unwired: 2 in, 2 out]
          }
          frame True {
            w391 = 0 ("Top Row")
            n253 = property on="CheckList" class="LstBox (strict)"() -> ("Number of Rows"=w393:u32)  [unwired: 2 in, 2 out]
            n254 = Initialize Array(0, w393) -> (w392:i32[])
            n255 = property on="CheckList" class="LstBox (strict)"("Top Row"=w391, "Value"=w391, "Item Symbols"=w392) -> ()  [unwired: 2 in, 2 out]
          }
        }
      }
      event "CheckList": Key Down {
        # "Update symbols on the listbox\nLeft and right keys check and uncheck"
        n256 = event-data() -> ("VKey"=w397:T22)  [unwired: 1 in]
        n257 = case shown="\"Left\", \"Right\"" w397 {
          selector: w397 -> [w402 _]
          tunnel: eventvkey."Left" ("VKey") -> [w400 _]
          frame "Left", "Right" {
            n258 = Equal?(x=w400, y=w402) -> (x = y?=w401:bool)
            n259 = Select(t=0, s=w401, f=1) -> (s? t:f=w403:i32)
            n260 = property on="CheckList" class="LstBox (strict)"() -> ("Item Symbols"=w406:i32[])  [unwired: 2 in, 2 out]
            n261 = Replace Array Subset(array=w406, new element=w403, index="CheckList") -> (w405:i32[])
            n262 = property on="CheckList" class="LstBox (strict)"("Item Symbols"=w405) -> ()  [unwired: 2 in, 2 out]
          }
          frame Default {
          }
        }
      }
      event "Motor.Enable": Value Change {
        # "When the test mode otor enable helper is set, update that\ntree row item's value"
        n263 = event-data() -> ("NewVal"=w412:bool)  [unwired: 1 in]
        n264 = Unbundle("Motor") -> ("Value"=w411:dbl)  [unwired: 1 out]
        n265 = Select(t=w411, s=w412, f=0.0) -> (s? t:f=w409:dbl)
        n266 = call <vilib>:"NT Write Number.vi"("Numeric"=w409, "Name"=w408) -> ()  [unwired: 9 in, 1 out]
      }
      event "Test Slider": Value Change {
        # "When the test mode slider helper is set, update that\ntree row item's value"
        n267 = event-data() -> ("NewVal"=w415:dbl)  [unwired: 1 in]
        n268 = call <vilib>:"NT Write Number.vi"("Numeric"=w415, "Name"=w416) -> ()  [unwired: 9 in, 1 out]
      }
      event "On/Off": Value Change {
        # "When the test mode on/off helper value is set, update that\ntree row item's value"
        n269 = event-data() -> ("NewVal"=w420:bool)  [unwired: 1 in]
        n270 = Boolean To (0,1)(Boolean=w420) -> (0, 1=w419:i16)
        n271 = call <vilib>:"NT Write Number.vi"("Numeric"=w419, "Name"=w418) -> ()  [unwired: 9 in, 1 out]
      }
      event "Rev/Fwd": Value Change {
        # "When the test mode helper value for relays is set, update that\ntree row item's value"
        n272 = event-data() -> ("NewVal.Forward"=w428:bool, "NewVal.Reverse"=w427:bool)  [unwired: 1 in]
        n273 = Boolean To (0,1)(Boolean=w428) -> (0, 1=w424:i16)
        n274 = Boolean To (0,1)(Boolean=w427) -> (0, 1=w426:i16)
        n275 = Negate(x=w426) -> (-x=w425:i16)
        n276 = Add(x=w424, y=w425) -> (x+y=w423:i16)
        n277 = call <vilib>:"NT Write Number.vi"("Numeric"=w423, "Name"=w422) -> ()  [unwired: 9 in, 1 out]
      }
      event "Test Ring": Value Change {
        # "When a test mode helper value is selected from the ring,\nset the tree item's variable to the string value"
        n278 = event-data() -> ("NewVal"=w432:u16)  [unwired: 1 in]
        n279 = property on="Test Ring" class="Ring (strict)"() -> ("Strings []"=w433:string[])  [unwired: 2 in, 2 out]
        n280 = Index Array(array=w433, index=w432) -> (element=w431:string)
        n281 = call <vilib>:"NT Write String.vi"("String"=w431, "Name"=w430) -> ()  [unwired: 9 in, 1 out]
      }
      event "Rec Mode": Value Change {
        # "Update globals for recording mode and path to read log from.\nClear when logging and let NetworkTables set path for vision to\nuse."
        n282 = event-data() -> ("NewVal"=w444:enum32{"Stop", "Record", "Playback"})  [unwired: 1 in]
        n283 = global write "WPI_DashboardLogging Global.vi" "Logging Filename"(path "") -> ()
        n284 = global write "WPI_DashboardLogging Global.vi" "Recording"(w444) -> ()
        n285 = case shown="\"Playback\"" w444 {
          tunnel: w443 -> [_ w446 w455]
          tunnel: [_ _ w454] -> w441
          tunnel: [_ _ w453] -> _
          tunnel: w439 -> [_ _ w451]
          tunnel: cluster{i32, i32} {-250, 170} -> [_ _ w450]
          tunnel: [_ _ T23 {"Image Size"=TRUE, "Image Type"=TRUE, "Pixel Value"=TRUE, "ROI Information"=TRUE, "Zoom Factor"=FALSE} ("Image Information Shown:All Elements")] -> w434
          tunnel: [_ _ TRUE ("Zoom Factor")] -> w435
          tunnel: w437 -> [_ _ w447]
          frame Default {
          }
          frame "Stop", "Record" {
            # "Place Window too"
            n286 = invoke class="VI" method="FP.Close"(reference=w446) -> (reference out=w445:refnum<vi>)  [unwired: 2 in, 2 out]
            n287 = invoke class="VI" method="Abort VI"(reference=w445) -> ()  [unwired: 2 in, 3 out]
          }
          frame "Playback" {
            n288 = call "Open Playback Panel.vi"("Offset"=w450, "DB VI Ref"=w451, "Playback in"=w455) -> ("Playback out"=w452:refnum<vi>)  [unwired: 8 in]
            n289 = register-events(w452, w447) -> (reference out=w454:refnum<event-registration>, error out=w453:errorcluster)  [unwired: 2 in]
          }
        }
        n290 = property on="Camera Image Right" class="ImageControl"("Image Information Shown"=w434, "Image Information Visible"=w435) -> ()  [unwired: 2 in, 2 out]
        n291 = property on="Camera Image" class="ImageControl"("Image Information Shown"=w434, "Image Information Visible"=w435) -> ()  [unwired: 2 in, 2 out]
        n292 = call <vilib>:"WPI_DashboardNT Log FieldName Cache.vi"("Operation"=enum16{"Lookup/Add", "Index", "Clear"}."Clear") -> ()  [unwired: 8 in, 3 out]
      }
      event Panel Close {
        w457 = enum32{"Stop", "Record", "Playback"}."Stop" ("Rec Mode")
        # "Playback window has been closed, abort"
        n293 = event-data() -> ()  [unwired: 1 in, 4 out]
        n294 = local write "Rec Mode"(w457) -> ()
        n295 = global write "WPI_DashboardLogging Global.vi" "Recording"(w457) -> ()
      }
      event Panel Close {
        # "Abort playback window and ourself"
        n296 = event-data() -> ()  [unwired: 1 in, 4 out]
        n297 = invoke class="VI" method="FP.Close"(reference=w461) -> (reference out=w460:refnum<vi>)  [unwired: 2 in, 2 out]
        n298 = invoke class="VI" method="Abort VI"(reference=w460) -> (error out=w459:errorcluster)  [unwired: 2 in, 2 out]
        n299 = invoke class="VI" method="Abort VI"(error in=w459) -> ()  [unwired: 2 in, 3 out]
      }
      event User Event {
        n300 = event-data() -> ("IDs"=w468:cluster{"RPC field ID":u16, "Unique ID":u16}, "String"=w467:string)  [unwired: 1 in]
        n301 = Bundle("IDs"=w468, "String"=w467) -> (w466:T9)  [unwired: 1 in]
        n302 = call <vilib>:"Retrieve RPC Response.vi"("RPC Response"=w466) -> ("Output"=w464:string[][])  [unwired: 10 in]
        n303 = Build Array (concatenate)(w462, w464) -> (w463:string[][])
        n304 = local write "Command Params"(w463) -> ()
        n305 = local write "Cmd Status"("" ("Cmd Status")) -> ()
      }
      event "Tree": Double Click {
        n306 = event-data() -> ("PlatMods"=w474:T26, "Tag"=w471:string)  [unwired: 1 in]
        n307 = Unbundle(w474) -> ("Shift"=w473:bool)  [unwired: 4 out]
        n308 = String Subset(string=w471, length (rest)=1 ("length (rest)")) -> (substring=w470:string)  [unwired: 1 in]
        n309 = Not(x=w473) -> (.not. x?=w472:bool)
        n310 = case shown="\"/\"" w470 {
          tunnel: w471 -> [_ w477]
          tunnel: w472 -> [_ w476]
          frame Default {
          }
          frame "/" {
            n311 = call <vilib>:"NT Update Persistence.vi"("Persistence"=w476, "Name"=w477) -> ()  [unwired: 9 in, 1 out]
          }
        }
      }
    }
  }
  n312 = while {
    tunnel: w65 -> [w479]
    i -> [w482]
    stop <- FALSE stop-if-true
    n313 = Wait (ms)(milliseconds to wait=u32 100) -> ()  [unwired: 1 out]
    n314 = case shown="\"Playback\"" "Rec Mode" {
      tunnel: w482 -> [_ _ w497]
      tunnel: [u32 2829099 ("Base Color") u32 11141120 ("Target Color") w486] -> w478
      frame "Stop", Default {
        # "Reset the color, extra updates don't cost much"
      }
      frame "Record" {
      }
      frame "Playback" {
        # "Playback"
        n315 = Quotient & Remainder(x=w497, y=u32 50 ("milliseconds to wait")) -> (x-y*floor(x/y)=w493:u32)  [unwired: 1 out]
        n316 = Divide(x=w493, y=u32 50 ("milliseconds to wait")) -> (x/y=w490:dbl)
        n317 = Multiply(x=6.283185307179586, y=w490) -> (x*y=w495:dbl)
        n318 = Sine(x=w495) -> (sin(x)=w494:dbl)
        n319 = Absolute Value(x=w494) -> (abs(x)=w487:dbl)
        n320 = call "Interpolate RGB Color.vi"("Proportion"=w487, "Target Color"=u32 30976, "Base Color"=u32 2829099) -> ("Result Color"=w486:u32)  [unwired: 8 in]
      }
    }
    n321 = property class="Pane"(reference=w479, "PaneColor"=w478) -> ()  [unwired: 1 in, 2 out]
  }
  n322 = local write "Dashboard Tab"(T2."Drive" ("Dashboard Tab")) -> ()
  n323 = property on="On/Off" class="Bool (strict)"("Visible"=w36) -> ()  [unwired: 2 in, 2 out]
  n324 = property on="Motor" class="Clust (strict)"("Visible"=w36) -> ()  [unwired: 2 in, 2 out]
  n325 = property on="Progress" class="Clust (strict)"("Visible"=w36) -> ()  [unwired: 2 in, 2 out]
  n326 = property on="Test Ring" class="Ring (strict)"("Visible"=w36) -> ()  [unwired: 2 in, 2 out]
  n327 = property on="Rev/Fwd" class="Clust (strict)"("Visible"=w36) -> ()  [unwired: 2 in, 2 out]
  n328 = while {
    tunnel: u16 1741 ("timeout ms (25000)") -> [w499]
    stop <- FALSE stop-if-true
    n329 = TCP Create Listener(10:w499) -> (0:w498:errorcluster, 3:w500:refnum<k5>)  [unwired: 4 in, 1 out]
    n330 = case shown="No Error" w498 {
      selector: w498 -> [w502 _]
      tunnel: w500 -> [w503 _]
      frame No Error {
        n331 = while {
          tunnel: w503 -> [w506]
          tunnel: w502 -> [w505]
          stop <- FALSE stop-if-true
          n332 = TCP Wait On Listener(8:w505, 11:w506) -> (0:w507:errorcluster, 4:w508:refnum<k5>)  [unwired: 2 in, 3 out]
          n333 = local write "TCP"(w508) -> ()
          n334 = case shown="No Error" w507 {
            frame No Error {
            }
            frame Error {
              n335 = Wait (ms)(milliseconds to wait=u32 1000) -> ()  [unwired: 1 out]
            }
          }
        }
      }
      frame Error {
        n336 = Wait (ms)(milliseconds to wait=u32 1000) -> ()  [unwired: 1 out]
      }
    }
  }
  n337 = local write "Command Selection"(u16 0 ("milliseconds to wait")) -> ()
  n338 = local write "Command Params"(string[][] [] ("Command Params")) -> ()
  n339 = global write "WPI_DashboardLogging Global.vi" "Recording"(w59) -> ()
  n340 = local write "Rec Mode"(w59) -> ()
  n341 = call <vilib>:"NT Write String.vi"("String"="Select Auto", "Name"="Auto Selector") -> ()  [unwired: 9 in, 1 out]
